vi "3.1-Wheel Setpoint Calibration.vi"() -> (0 "Array":i32[](array[numeric]))   [LabVIEW 2010]
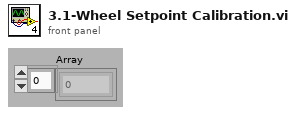
[diagram p1: front panel]
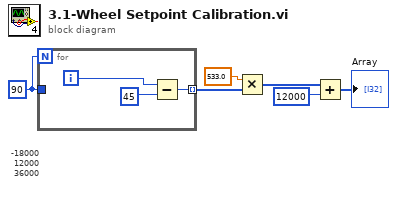
[diagram p0: block diagram]
diagram:
  w5 = 90
  # "-18000\n 12000\n 36000"
  n1 = for {
    N: w5 -> [_]
    tunnel: [w8] -> w4 mode=indexing
    tunnel: w5 -> [_]
    i -> [w7]
    n2 = Subtract(x=w7, y=45) -> (x-y=w8:i32)
  }
  n3 = Multiply(x=533.0 ("ticks per degree"), y=w4) -> (x*y=w2:i32[])
  n4 = Add(x=w2, y=12000 ("magic zero point number")) -> (x+y=→"Array":i32[])
